vi "sub_lidar_graph.vi"() -> (2 "max pnt":u16)   [LabVIEW 2019]
uses:
  Ctrl/obstacle_info.ctl
panel:
  out "each_arr_size":i32
  out "x > y?":bool
  out "n_4":i32
  out "all_arr_size":i32
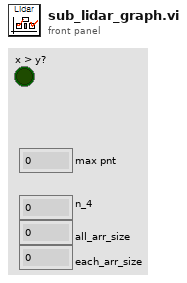
[diagram p1: front panel]
types:
  T1 = typedef "obstacle_info.ctl" = enum16{"init", "read", "obstacle status in", "write limit", "inrange pt-n"}
  T2 = cluster{"VLP16 cfg":refnum<vi>, "TIM571 cfg":refnum<vi>, "PID cfg":refnum<vi>, "AGV cfg":refnum<vi>, "GNSS cfg":refnum<vi>, "camera cfg":refnum<vi>, "ybbaek copyright":refnum<vi>, "Obstacle limit cfg":refnum<vi>, "State machine cfg":refnum<vi>, "Lookahead cfg":refnum<vi>, "waypoint files cfg":refnum<vi>, "Vison cfg":refnum<vi>, "RPLidar cfg":refnum<vi>, "point all":refnum<vi>, "HW info":refnum<vi>, "Joystick cfg":refnum<vi>, "GMapControl":refnum<vi>, "IMU cfg":refnum<vi>, "ledmatrix cfg":refnum<vi>}
  T3 = cluster{"h range":cluster{i16, i16}, "v range":cluster{i8, i8}, "bounding box arr":cluster{"X":dbl, "Y":dbl, "W":dbl, "H":dbl}[]}
  T4 = cluster{"Array out":cluster{"x":dbl, "y":dbl}[]}[]
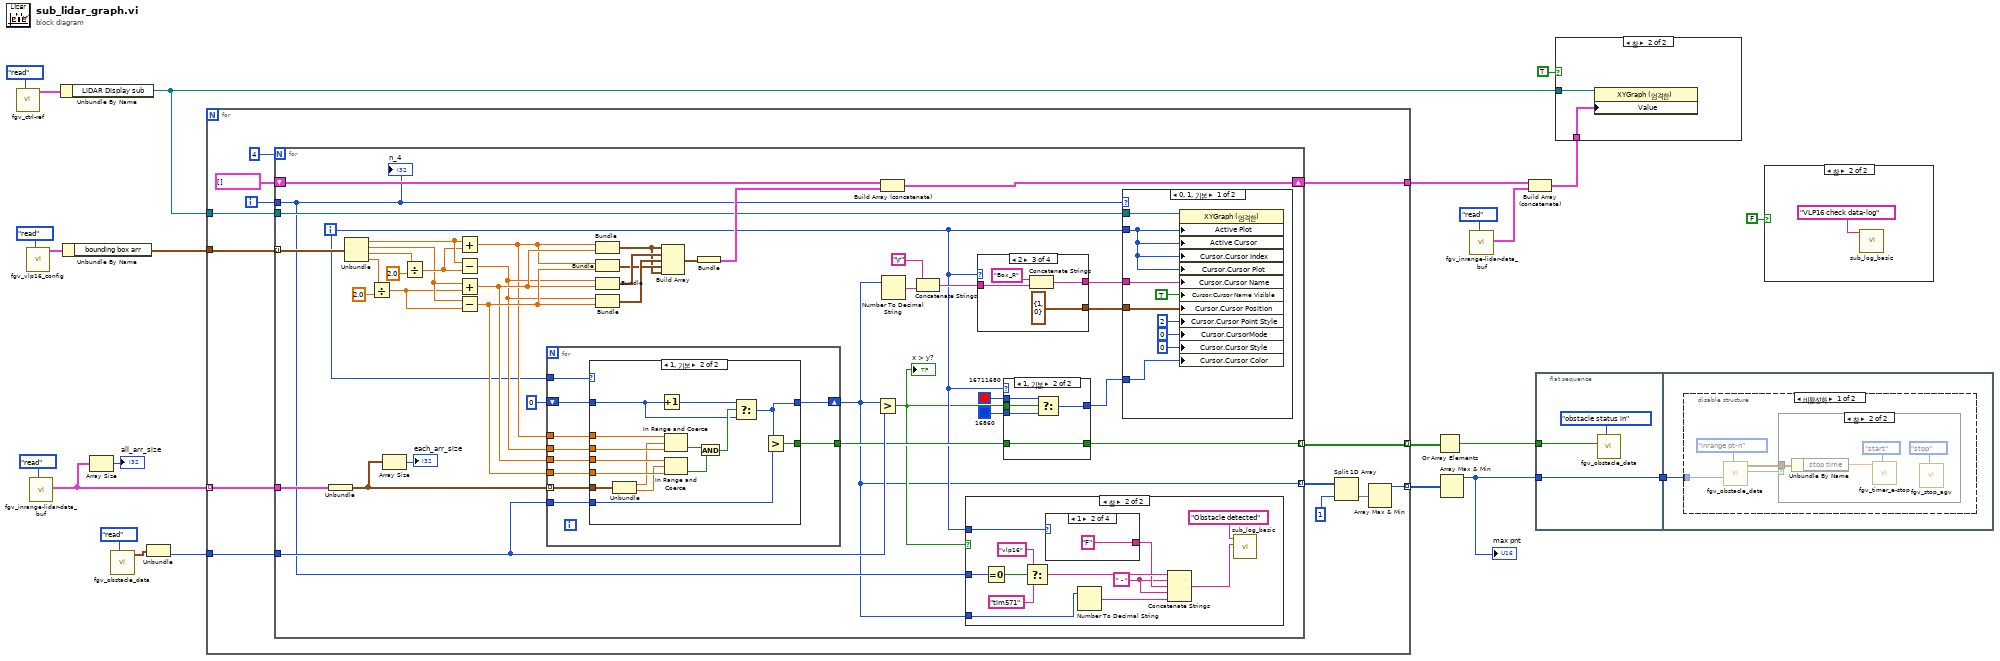
[diagram p0: block diagram]
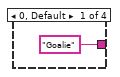
[diagram p7: hidden frame]
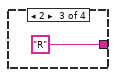
[diagram p8: hidden frame]
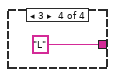
[diagram p9: hidden frame]
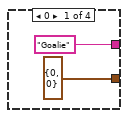
[diagram p11: hidden frame]
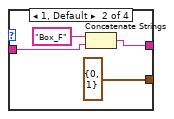
[diagram p12: hidden frame]
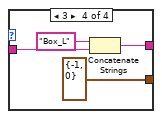
[diagram p13: hidden frame]
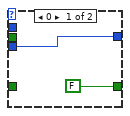
[diagram p14: hidden frame]
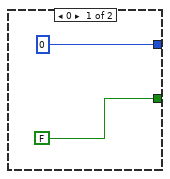
[diagram p15: hidden frame]
diagram:
  n1 = call "fgv_ctrl-ref.vi"("cmd"=enum16{"write", "read"}."read") -> ("ref 2"=w21:T2)  [unwired: 9 in, 1 out]
  n2 = call "fgv_vlp16_config.vi"("cmd"=enum16{"read", "write"}."read") -> ("VLP16 cfg out"=w19:T3)  [unwired: 10 in]
  n3 = call "fgv_inrange-lidar-data_buf.vi"("cmd"=enum16{"read", "write"}."read") -> ("in range data new out"=w7:T4)  [unwired: 9 in, 1 out]
  n4 = Unbundle By Name(w21) -> ("LiDAR Display sub"=w16:refnum<vi>)
  n5 = Unbundle By Name(w19) -> ("bounding box arr"=w18:cluster{"X":dbl, "Y":dbl, "W":dbl, "H":dbl}[])
  n6 = Array Size(array=w7) -> (size(s)=→"all_arr_size":i32)
  n7 = call "fgv_obstacle_data.vi"("cmd"=obstacle_info."read") -> ("limit out"=w5:cluster{"RL range":dbl, "Point limit":u16})  [unwired: 7 in, 3 out]
  n8 = Unbundle(w5) -> ("Point limit"=w3:u16)  [unwired: 1 out]
  n9 = for {
    tunnel: w18 -> [w32]
    tunnel: w16 -> [w35]
    tunnel: [w34] -> w13
    tunnel: w7 -> [w33] mode=indexing
    tunnel: [w30] -> w14 mode=indexing
    tunnel: [w29] -> w11 mode=indexing
    tunnel: w3 -> [w24]
    i -> [w25]
    n10 = for {
      N: 4 -> [_]
      tunnel: w32 -> [w61] mode=indexing
      shift-right: [w69] -> w34
      shift-left: cluster{cluster{dbl, dbl}[]}[] [] -> [w68]
      tunnel: w35 -> [w60]
      tunnel: w33 -> [w54]
      tunnel: [w51] -> w30 mode=indexing
      tunnel: [w37] -> w28 mode=indexing
      tunnel: w25 -> [w38]
      tunnel: w24 -> [w42]
      i -> [w40]
      n11 = Unbundle(w54) -> ("Array out"=w43:cluster{"x":dbl, "y":dbl}[])
      n12 = Unbundle(w61) -> ("X"=w73:dbl, "Y"=w63:dbl, "W"=w77:dbl, "H"=w74:dbl)
      n13 = Divide(x=w74, y=2.0) -> (x/y=w62:dbl)
      n14 = Array Size(array=w43) -> (size(s)=→"each_arr_size":i32)
      n15 = Divide(x=w77, y=2.0) -> (x/y=w72:dbl)
      n16 = Add(x=w73, y=w72) -> (x+y=w56:dbl)
      n17 = Subtract(x=w73, y=w72) -> (x-y=w57:dbl)
      n18 = Add(x=w63, y=w62) -> (x+y=w58:dbl)
      n19 = Subtract(x=w63, y=w62) -> (x-y=w59:dbl)
      n20 = for {
        tunnel: w59 -> [w133]
        tunnel: w58 -> [w132]
        tunnel: w57 -> [w131]
        tunnel: w56 -> [w130]
        tunnel: w43 -> [w129] mode=indexing
        shift-right: [w127] -> w37
        shift-left: 0 -> [w128]
        tunnel: [w124] -> w41
        tunnel: w40 -> [w126]
        tunnel: w42 -> [w125]
        n21 = case shown="1, 기본" w126 {
          tunnel: w133 -> [_ w150]
          tunnel: w132 -> [_ w149]
          tunnel: w131 -> [_ w148]
          tunnel: w130 -> [_ w147]
          tunnel: w129 -> [_ w146]
          tunnel: w128 -> [_ w139]
          tunnel: [0 w138] -> w127
          tunnel: w125 -> [_ w137]
          tunnel: [FALSE w136] -> w124
          frame 0 {
          }
          frame 1, Default {
            n22 = Unbundle(w146) -> ("x"=w145:dbl, "y"=w144:dbl)
            n23 = Increment(x=w139) -> (x+1=w140:i32)
            n24 = In Range and Coerce(upper limit=w147, x=w145, lower limit=w148) -> (In Range?=w143:bool)  [unwired: 1 out]
            n25 = In Range and Coerce(upper limit=w149, x=w144, lower limit=w150) -> (In Range?=w142:bool)  [unwired: 1 out]
            n26 = And(x=w143, y=w142) -> (x .and. y?=w141:bool)
            n27 = Select(t=w140, s=w141, f=w139) -> (s? t:f=w138:i32)
            n28 = Greater?(x=w138, y=w137) -> (0:w136:bool)
          }
        }
      }
      n29 = Bundle(w56, w58) -> (w64:cluster{dbl, dbl})  [unwired: 1 in]
      n30 = Bundle(w56, w59) -> (w65:cluster{dbl, dbl})  [unwired: 1 in]
      n31 = Bundle(w57, w58) -> (w67:cluster{dbl, dbl})  [unwired: 1 in]
      n32 = Bundle(w57, w59) -> (w66:cluster{dbl, dbl})  [unwired: 1 in]
      n33 = Build Array(w64, w67, w66, w65, w64) -> (w71:cluster{dbl, dbl}[])
      n34 = Bundle(w71) -> (w70:cluster{cluster{dbl, dbl}[]})  [unwired: 1 in]
      n35 = Greater?(x=w37, y=w42) -> (0:w39:bool)
      "x > y?" <- w39
      n36 = Build Array (concatenate)(w68, w70) -> (w69:cluster{cluster{dbl, dbl}[]}[])
      n37 = Number To Decimal String(number=w37) -> (decimal integer string=w50:string)  [unwired: 1 in]
      n38 = Concatenate Strings("\r", w50) -> (w48:string)
      n39 = case shown="참" w39 {
        tunnel: w38 -> [_ w88]
        tunnel: w40 -> [_ w83]
        tunnel: w37 -> [_ w78]
        frame False {
        }
        frame True {
          w80 = " - " ("문자열")
          n40 = Equal To 0?(x=w88) -> (x = 0?=w87:bool)
          n41 = Select(t="vlp16" ("Title"), s=w87, f="tim571" ("Title")) -> (s? t:f=w84:string)
          n42 = case shown="1" w83 {
            tunnel: ["Goalie" ("Title") "F" ("Title") "R" ("Title") "L" ("Title")] -> w82
            frame 0, Default {
            }
            frame 1 {
            }
            frame 2 {
            }
            frame 3 {
            }
          }
          n43 = Number To Decimal String(number=w78) -> (decimal integer string=w79:string)  [unwired: 1 in]
          n44 = Concatenate Strings(w84, w80, w82, w80, w79) -> (w81:string)
          n45 = call "sub_log_basic.vi"("desc"=w81, "Title"="Obstacle detected") -> ()  [unwired: 9 in, 1 out]
        }
      }
      n46 = case shown="2" w40 {
        tunnel: ["Goalie" ("문자열") w106 w110 w114] -> w45
        tunnel: w48 -> [_ w105 w111 w115]
        tunnel: [cluster{i16, i16} {0, 0} cluster{i16, i16} {0, 1} cluster{i16, i16} {1, 0} cluster{i16, i16} {-1, 0}] -> w46
        frame 0 {
        }
        frame 1, Default {
          n47 = Concatenate Strings("Box_F" ("문자열"), w105) -> (w106:string)
        }
        frame 2 {
          n48 = Concatenate Strings("Box_R" ("문자열"), w111) -> (w110:string)
        }
        frame 3 {
          n49 = Concatenate Strings("Box_L" ("문자열"), w115) -> (w114:string)
        }
      }
      n50 = case shown="1, 기본" w40 {
        tunnel: w39 -> [_ w120]
        tunnel: [w118 w123] -> w47
        tunnel: u32 16711680 -> [_ w122]
        tunnel: u32 16860 -> [w118 w121]
        tunnel: w41 -> [_ w119]
        tunnel: [FALSE w119] -> w51
        frame 0 {
        }
        frame 1, Default {
          n51 = Select(t=w122, s=w120, f=w121) -> (s? t:f=w123:u32)
        }
      }
      n52 = case shown="0, 1, 기본" w38 {
        tunnel: w60 -> [w100 _]
        tunnel: w40 -> [w97 _]
        tunnel: w47 -> [w96 _]
        tunnel: w46 -> [w95 _]
        tunnel: w45 -> [w94 _]
        frame 0, 1, Default {
          n53 = property on="프로퍼티 노드" class="XYGraph (엄격한)"(reference=w100, "Active Plot"=w97, "Active Cursor"=w97, "Cursor.Cursor Index"=w97, "Cursor.Cursor Plot"=w97, "Cursor.Cursor Name"=w94, "Cursor.Cursor Name Visible"=TRUE ("커서.커서 이름 보이기"), "Cursor.Cursor Position"=w95, "Cursor.Cursor Point Style"=u8 2 ("커서.커서 포인트 스타일"), "Cursor.CursorMode"=u32 0 ("커서.커서 모드"), "Cursor.Cursor Style"=u8 0 ("커서.커서 스타일"), "Cursor.Cursor Color"=w96) -> ()  [unwired: 1 in, 2 out]
        }
        frame 22 {
        }
      }
      "n_4" <- w38
    }
    n54 = Split 1D Array(array=w28, index=1 ("인덱스")) -> (second subarray=w26:i32[])  [unwired: 1 out]
    n55 = Array Max & Min(array=w26) -> (max value=w29:i32)  [unwired: 3 out]
  }
  n56 = Or Array Elements(Boolean array=w14) -> (logical OR=w2:bool)
  n57 = Array Max & Min(array=w11) -> (max value=w9:i32)  [unwired: 3 out]
  "max pnt" <- w9
  n58 = call "fgv_inrange-lidar-data_buf.vi"("cmd"=enum16{"read", "write"}."read") -> ("in range data new out"=w12:T4)  [unwired: 9 in, 1 out]
  n59 = Build Array (concatenate)(w13, w12) -> (w17:T4)
  n60 = flat-sequence {
    tunnel: w2 -> [w152]
    tunnel: [w151] -> w10
    tunnel: w9 -> [w151]
    tunnel: w10 -> [w154]
    frame #0 {
      n61 = call "fgv_obstacle_data.vi"("cmd"=obstacle_info."obstacle status in", "obstacle in"=w152) -> ()  [unwired: 6 in, 4 out]
    }
    frame #1 {
      n62 = disable-structure shown="비활성화" {
        disable-tunnel: w154 -> [w157 _]
        frame Disabled {
          n63 = call "fgv_obstacle_data.vi"("cmd"=obstacle_info."inrange pt-n", "inrange pt-n"=w157) -> ("obstacle out"=w156:bool, "limit out"=w155:cluster{"RL range":dbl, "Point limit":u16})  [unwired: 6 in, 2 out]
          n64 = case shown="참" w156 {
            tunnel: w155 -> [_ w160]
            frame False {
            }
            frame True {
              n65 = Unbundle By Name(w160) -> ("stop time"=w159:dbl)
              n66 = call "fgv_timer_e-stop.vi"("cmd"=enum16{"check", "start", "pause"}."start", "target time"=w159) -> ()  [unwired: 7 in, 3 out]
              n67 = call "fgv_stop_agv.vi"("cmd"=enum16{"ini", "read", "stop"}."stop") -> ()  [unwired: 10 in, 1 out]
            }
          }
        }
        frame Enabled {
        }
      }
    }
  }
  n68 = case shown="참" TRUE {
    tunnel: w17 -> [_ w164]
    tunnel: w16 -> [_ w163]
    frame False {
    }
    frame True {
      n69 = property class="XYGraph (엄격한)"(reference=w163, "Value"=w164) -> ()  [unwired: 1 in, 2 out]
    }
  }
  n70 = case shown="참" FALSE {
    frame False {
    }
    frame True {
      n71 = call "sub_log_basic.vi"("Title"="VLP16 check data-log") -> ()  [unwired: 10 in, 1 out]
    }
  }
